vi "Add XML Dependency.vi"(8 "error in (no error)":errorcluster, 10 "Dependency Parameters":T1, 11 "Project XML Editor in":refnum<class "Project XML Editor.lvclass">) -> (0 "error out":errorcluster, 3 "Project XML Editor out":refnum<class "Project XML Editor.lvclass">)   [LabVIEW 2018, in ".LVLIBP CD XML Updater.lvlib" / "Project XML Editor.lvclass"]
uses:
  Project XML Editor.lvclass
  TypeDefs/Dependency Parameters.ctl
  Project XML Editor.lvclass/Project XML Editor.ctl
  <vilib>/xml/Close Reference(Node).vi
  <resource>/objmgr/DOMUserDefRef.rc
  <vilib>/xml/NI_XML.lvlib
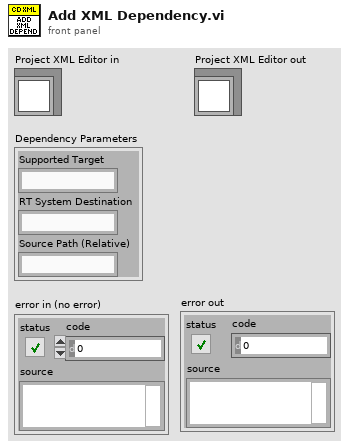
[diagram p1: front panel]
types:
  T1 = typedef ".LVLIBP CD XML Updater.lvlib/Project XML Editor.lvclass/Dependency Parameters.ctl" = cluster{"Supported Target":string, "RT System Destination":string, "Source Path (Relative)":string}
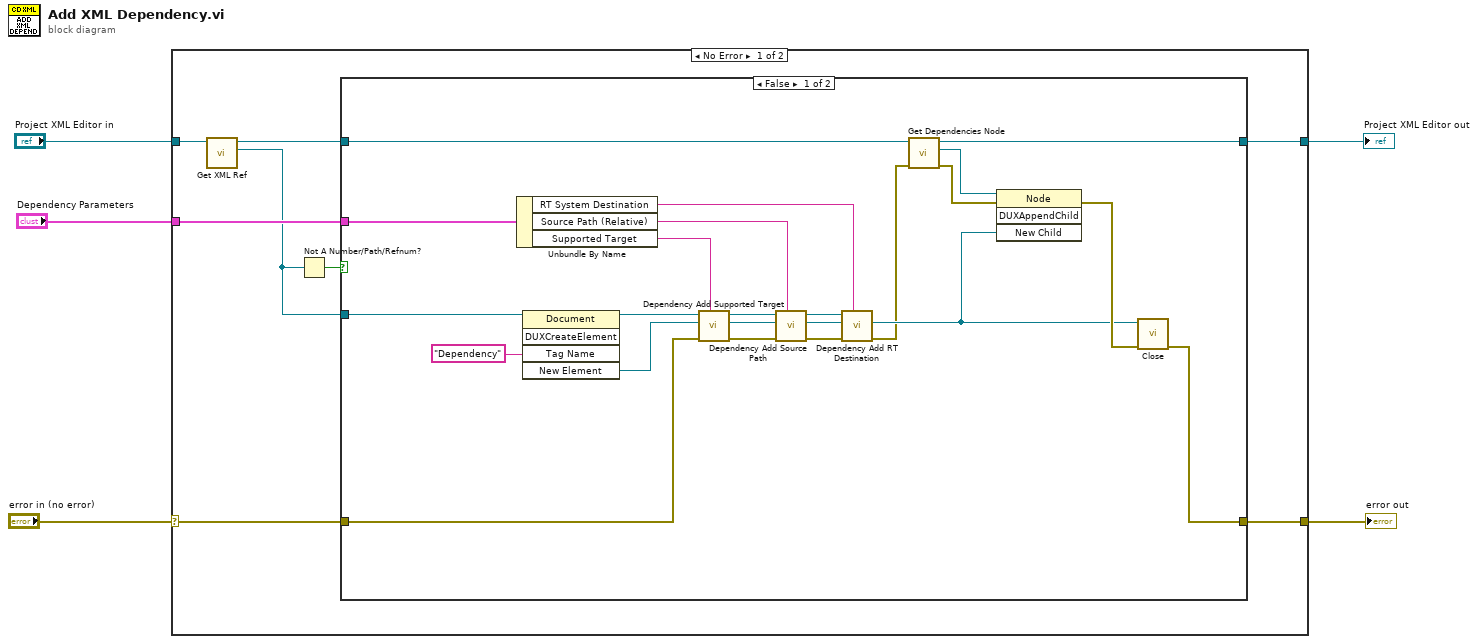
[diagram p0: block diagram]
diagram:
  n1 = case shown="No Error" "error in (no error)" {
    selector: "error in (no error)" -> [w9 w40]
    tunnel: "Project XML Editor in" -> [w13 w39]
    tunnel: [w12 w40] -> w4
    tunnel: [w11 w39] -> w3
    tunnel: "Dependency Parameters" -> [w8 _]
    frame No Error {
      n2 = call "Get XML Ref.vi"("Project XML Editor in"=w13) -> ("XML Ref"=w7:refnum<k20>, "Project XML Editor out"=w10:refnum<class "Project XML Editor.lvclass">)  [unwired: 9 in]
      n3 = Not A Number/Path/Refnum?(number/path/refnum=w7) -> (NaN/Path/Refnum?=w6:bool)
      n4 = case shown="False" w6 {
        tunnel: [w36 w38] -> w12
        tunnel: [w32 w37] -> w11
        tunnel: w10 -> [w30 w37]
        tunnel: w9 -> [w18 w38]
        tunnel: w8 -> [w17 _]
        tunnel: w7 -> [w14 _]
        frame False {
          n5 = Unbundle By Name(w17) -> ("RT System Destination"=w22:string, "Source Path (Relative)"=w25:string, "Supported Target"=w28:string)
          n6 = invoke class="Document" method="DUXCreateElement"(reference=w14, "Tag Name"="Dependency") -> (reference out=w33:refnum<k20>, "New Element"=w34:refnum<k20>)  [unwired: 3 in, 3 out]
          n7 = call "Dependency Add Supported Target.vi"("Supported Target Value"=w28, "error in (no error)"=w18, "Dependency ref in"=w34, "XML File ref in"=w33) -> ("error out"=w20:errorcluster, "Dependency ref out"=w27:refnum<k20>, "XML File ref out"=w26:refnum<k20>)  [unwired: 5 in]
          n8 = call "Dependency Add Source Path.vi"("Source Path (relative)"=w25, "error in (no error)"=w20, "Dependency ref in"=w27, "XML File ref in"=w26) -> ("error out"=w19:errorcluster, "Dependency ref out"=w23:refnum<k20>, "XML File ref out"=w24:refnum<k20>)  [unwired: 5 in]
          n9 = call "Dependency Add RT Destination.vi"("Supported Target Value"=w22, "error in (no error)"=w19, "Dependency ref in"=w23, "XML File ref in"=w24) -> ("error out"=w16:errorcluster, "Dependency ref out"=w21:refnum<k20>)  [unwired: 5 in, 1 out]
          n10 = call "Get Dependencies Node.vi"("error in (no error)"=w16, "Project XML Editor in"=w30) -> ("error out"=w15:errorcluster, "Dependencies out"=w31:refnum<k20>, "Project XML Editor out"=w32:refnum<class "Project XML Editor.lvclass">)  [unwired: 6 in, 1 out]
          n11 = invoke class="Node" method="DUXAppendChild"(reference=w31, error in=w15, "New Child"=w21) -> (error out=w35:errorcluster)  [unwired: 1 in, 3 out]
          n12 = call-poly <vilib>:"Close.vi"("error in (no error)"=w35, "node"=w21) -> ("error out"=w36:errorcluster)  [unwired: 7 in]
        }
        frame True {
        }
      }
    }
    frame Error {
    }
  }
  "error out" <- w4
  "Project XML Editor out" <- w3
